vi "SGUI Set Boolean State By Label.vi"(5 "generate error if not found? (True)":bool=TRUE, 7 "binary state in (False)":bool, 10 "error in":errorcluster, 11 "control label(s) ('btn stop')":string="btn stop") -> (2 "error out":errorcluster, 3 "found and type matches?":bool)   [LabVIEW 2013, in "varilib.lvlib"]
doc: "Sets state of one or multiple boolean controls designated by its label name. The references and labels must be first registered by calling 'SGUI Register Controls'. If not found or not a boolean type, it will by default return error however it ignores input error (executes anyway)."
uses:
  varilib.lvlib
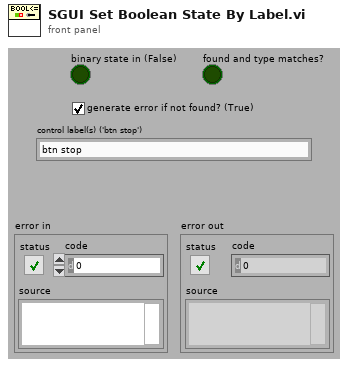
[diagram p1: front panel]
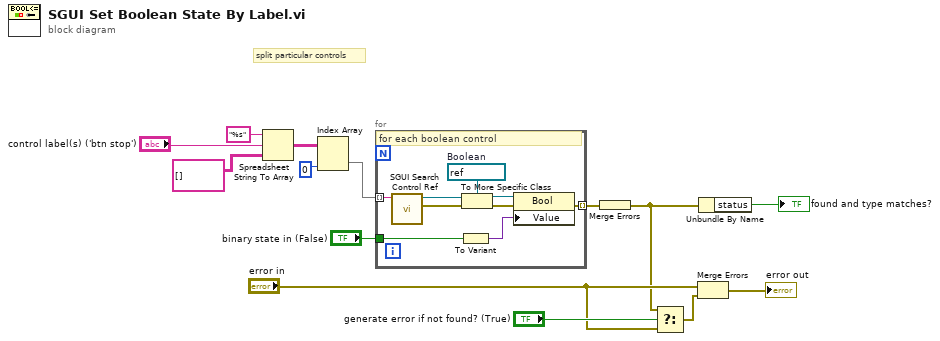
[diagram p0: block diagram]
diagram:
  # "split particular controls"
  n1 = Spreadsheet String To Array(format string="%s", spreadsheet string="control label(s) ('btn stop')", array type (2D Dbl)=string[][] []) -> (array=w7:string[][])  [unwired: 1 in]
  n2 = Index Array(array=w7, index (col)=0 ("disabled index (col)")) -> (element=w2:string[])  [unwired: 1 in]
  n3 = for {
    tunnel: "binary state in (False)" -> [w17]
    tunnel: w2 -> [w16] mode=indexing
    tunnel: [w15] -> w9 mode=indexing
    w19 = refnum<vi> refnum  # Boolean
    # "for each boolean control"
    n4 = call "SGUI Search Control Ref.vi"("control label (empty)"=w16) -> ("error out"=w23:errorcluster, "control ref out"=w22:refnum<vi>)  [unwired: 8 in, 1 out]
    n5 = To Variant(anything=w17) -> (Variant=w18:variant)
    n6 = To More Specific Class(target class=w19, reference=w22, error in=w23) -> (specific class reference=w20:refnum<vi>, error out=w21:errorcluster)
    n7 = property class="Bool"(reference=w20, error in=w21, "Value"=w18) -> (error out=w15:errorcluster)  [unwired: 1 out]
  }
  n8 = Merge Errors(w9) -> (w1:errorcluster)
  n9 = Select(t=w1, s="generate error if not found? (True)", f="error in") -> (s? t:f=w11:errorcluster)
  n10 = Merge Errors("error in", w11) -> (→"error out":errorcluster)
  n11 = Unbundle By Name(w1) -> ("status"=→"found and type matches?":bool)
